vi "Config Frequency Channel.vi"(0 "VISA Resource Name":refnum<visa-resource-name>, 5 "State (F: OFF)":bool, 7 "Channel Band (0: Standard Base)":T1(ring), 9 "Channel Number (1)":i32=1, 11 "error in (no error)":errorcluster {"code" format="%.0x"}) -> (4 "VISA Resource Name Out":refnum<visa-resource-name>, 15 "error out":errorcluster {"code" format="%.0x"})   [LabVIEW 2012, in "Agilent ESG Series.lvlib"]
doc: "This VI configures frequency channels parameters.\n\nNotes:\n(1) This VI is supported for Agilent E4438C only."
uses:
  <instrlib>/Agilent ESG Series/Agilent ESG Series.lvlib
panel:
  # "ON"
  # "OFF"
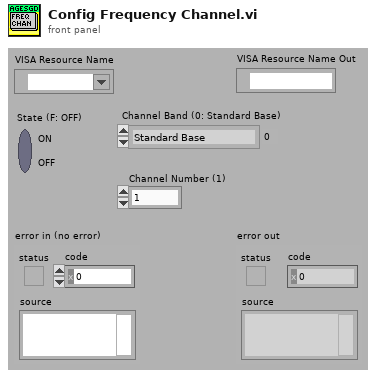
[diagram p1: front panel]
types:
  T1 = enum16{"Standard Base", "Standard Mobile", "P-Gsm 900 Base", "P-Gsm 900 Mobile", "E-Gsm 900 Base", "E-Gsm 900 Mobile", "R-Gsm 900 Base", "R-Gsm 900 Mobile", "DCS 1800 Base", "DCS 1800 Mobile", "PCS 1900 Base", "PCS 1900 Mobile", "Gsm 450 Base", "Gsm 450 Mobile", "Gsm 480 Base", "Gsm 480 Mobile", "Gsm 850 Base", "Gsm 850 Mobile", "800MHz Base", "800MHz Mobile", "1500MHz Base", "1500MHz Mobile", "Base 390-400", "Base 420-430", "Base 460-470", "Base 915-921", "Mobile 380-390", "Mobile 410-420", "Mobile 450-460", "Mobile 870-876", "Standard PHS", "Standard DECT"}
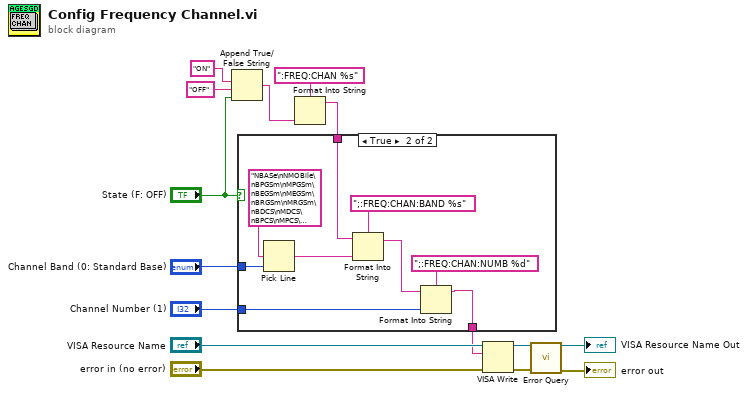
[diagram p0: block diagram]
diagram:
  n1 = Append True/False String(1:"State (F: OFF)", 2:"OFF" ("false string"), 3:"ON" ("multi-line string")) -> (0:w2:string)  [unwired: 1 in]
  n2 = Format Into String(format string=":FREQ:CHAN %s", w2) -> (resulting string=w4:string)  [unwired: 2 in, 1 out]
  n3 = case shown="True" "State (F: OFF)" {
    tunnel: "Channel Band (0: Standard Base)" -> [_ w25]
    tunnel: "Channel Number (1)" -> [_ w20]
    tunnel: w4 -> [w16 w18]
    tunnel: [w16 w17] -> w3
    frame False {
    }
    frame True {
      n4 = Pick Line(multi-line string="NBASe\nNMOBile\nBPGSm\nMPGSm\nBEGSm\nMEGSm\nBRGSm\nMRGSm\nBDCS\nMDCS\nBPCS\nMPCS\nB450\nGM450\nB480\nM480\nB850\nM850\nB8\nM8\nB15\nM15\nB390\nB420\nB460\nB915\nM380\nM410\nM450\nM870\nPHS\nDECT", line index=w25) -> (output string=w23:string)  [unwired: 1 in]
      n5 = Format Into String(format string=";:FREQ:CHAN:BAND %s", initial string=w18, w23) -> (resulting string=w19:string)  [unwired: 1 in, 1 out]
      n6 = Format Into String(format string=";:FREQ:CHAN:NUMB %d", initial string=w19, w20) -> (resulting string=w17:string)  [unwired: 1 in, 1 out]
    }
  }
  n7 = VISA Write(VISA resource name="VISA Resource Name", write buffer=w3, error in (no error)="error in (no error)") -> (VISA resource name out=w11:refnum<visa-resource-name>, error out=w10:errorcluster)  [unwired: 1 out]
  n8 = call <instrlib>:"Error Query.vi"("VISA Resource Name"=w11, "error in (no error)"=w10) -> ("VISA Resource Name Out"=→"VISA Resource Name Out":refnum<visa-resource-name>, "error out"=→"error out":errorcluster)  [unwired: 10 in, 2 out]
